vi "Write GPIB Addr.vi"(8 "error in (no error)":errorcluster, 10 "GPIB Addr":refnum<visa-resource-name>, 11 "SR 3XX HVPS in":refnum<class "SR 3XX HVPS.lvclass">) -> (0 "error out":errorcluster, 3 "SR 3XX HVPS out":refnum<class "SR 3XX HVPS.lvclass">)   [LabVIEW 2013, in "SR 3XX HVPS.lvclass"]
uses:
  SR 3XX HVPS.lvclass
  SR 3XX HVPS.lvclass/SR 3XX HVPS.ctl
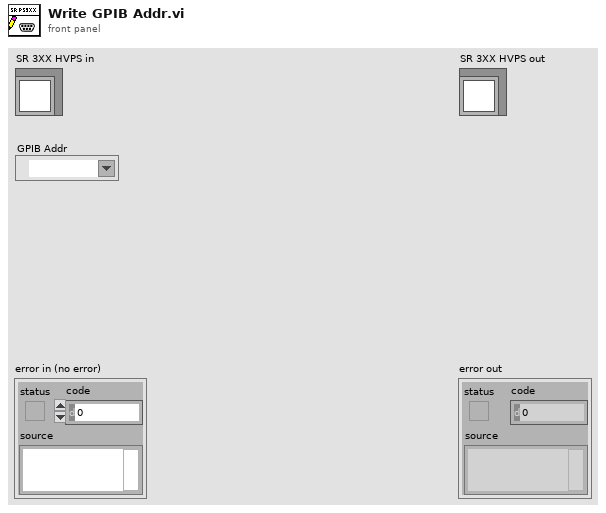
[diagram p1: front panel]
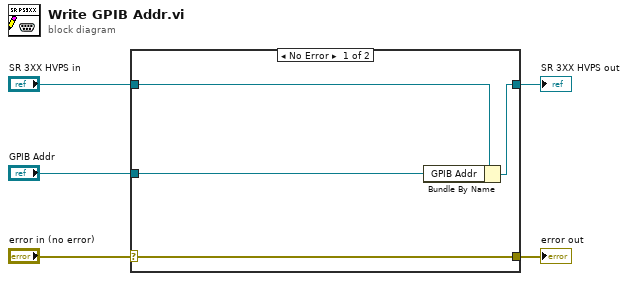
[diagram p0: block diagram]
diagram:
  n1 = case shown="No Error" "error in (no error)" {
    selector: "error in (no error)" -> [w9 w10]
    tunnel: [w9 w10] -> w4
    tunnel: [w7 w11] -> w2
    tunnel: "SR 3XX HVPS in" -> [w8 w11]
    tunnel: "GPIB Addr" -> [w6 _]
    frame No Error {
      n2 = Bundle By Name(cluster=w8, "GPIB Addr"=w6) -> (w7:refnum<class "SR 3XX HVPS.lvclass">)
    }
    frame Error {
    }
  }
  "error out" <- w4
  "SR 3XX HVPS out" <- w2
